vi "Load Player Types.vi"(8 "error in":errorcluster, 11 "Reversi in":refnum<class "Reversi.lvclass">) -> (0 "error out":errorcluster, 3 "Reversi out":refnum<class "Reversi.lvclass">)   [LabVIEW 2020, in "Reversi.lvlib" / "Reversi.lvclass"]
uses:
  Reversi.lvclass
  Player/Player.lvclass
  Reversi.lvclass/Reversi.ctl
  NonOOPlayer/NonOOPlayer.lvclass
  J:/Code/Reversi/Reversi/Player/Player.lvclass
  Human/Human.lvclass
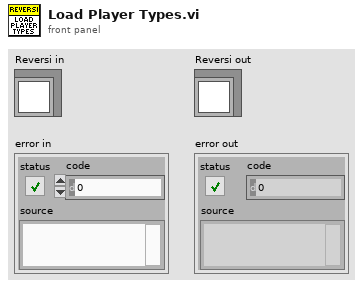
[diagram p1: front panel]
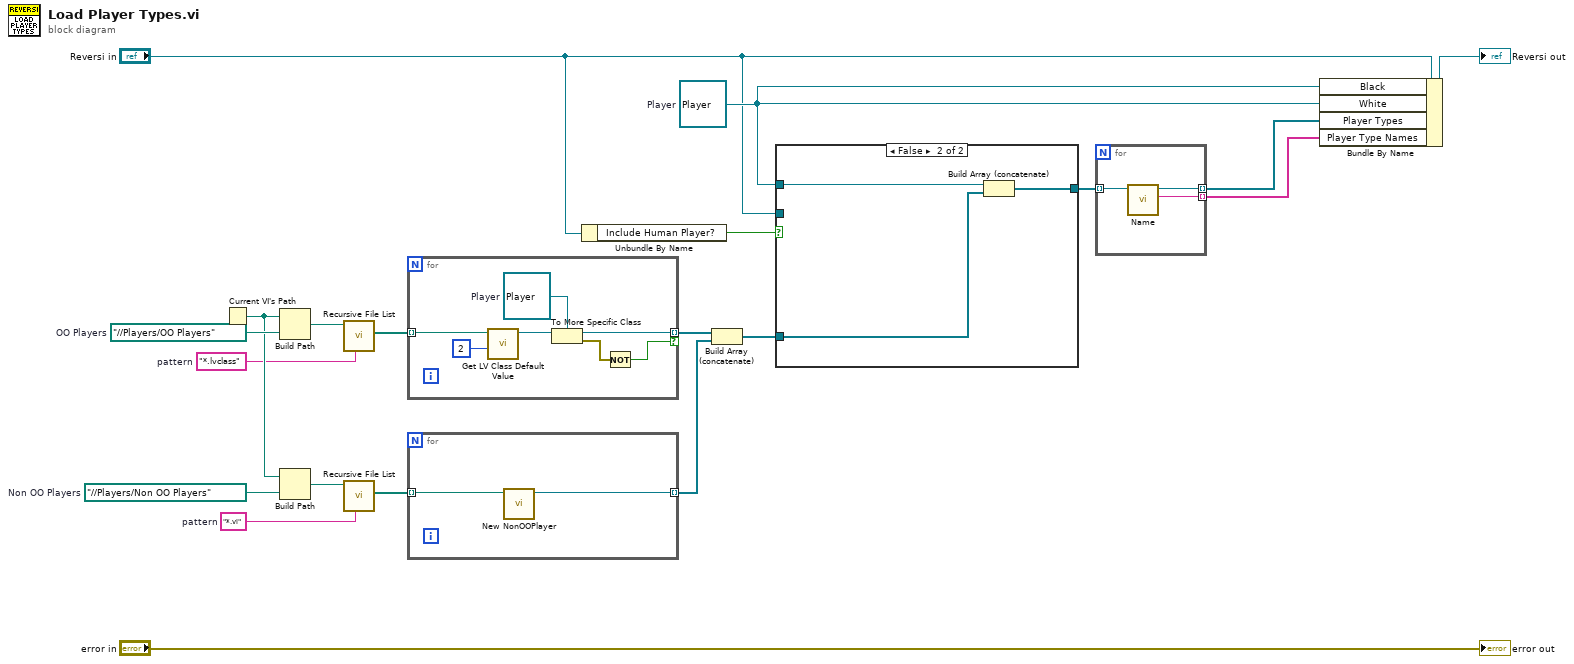
[diagram p0: block diagram]
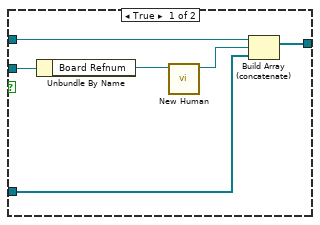
[diagram p2: hidden frame]
diagram:
  w9 = "*.vi"  # pattern
  w10 = "*.lvclass"  # pattern
  w13 = path "../../Players/Non OO Players"  # Non OO Players
  w14 = path "../../Players/OO Players"  # OO Players
  w17 = refnum<class "Player.lvclass"> refnum  # Player
  n1 = Current VI's Path() -> (path=w12:path)
  n2 = Build Path(base path=w12, name or relative path=w14) -> (appended path=w11:path)
  n3 = Build Path(base path=w12, name or relative path=w13) -> (appended path=w8:path)
  n4 = call <vilib>:"Recursive File List.vi"("pattern"=w10, "Folder Path"=w11) -> ("All Files in Dir"=w7:path[])  [unwired: 5 in, 4 out]
  n5 = call <vilib>:"Recursive File List.vi"("pattern"=w9, "Folder Path"=w8) -> ("All Files in Dir"=w6:path[])  [unwired: 5 in, 4 out]
  n6 = for {
    tunnel: w7 -> [w26] mode=indexing
    tunnel: [w22] -> w5 mode=indexing if=w21
    w23 = refnum<class "Player.lvclass"> refnum  # Player
    n7 = call <vilib>:"Get LV Class Default Value.vi"("options"=u32 2, "class path"=w26) -> ("object"=w24:refnum<class>)  [unwired: 8 in, 1 out]
    n8 = To More Specific Class(target class=w23, reference=w24) -> (specific class reference=w22:refnum<class "Player.lvclass">, error out=w27:errorcluster)  [unwired: 1 in]
    n9 = Not(x=w27) -> (.not. x?=w21:bool)
  }
  n10 = for {
    tunnel: w6 -> [w29] mode=indexing
    tunnel: [w28] -> w4 mode=indexing
    n11 = call "New NonOOPlayer.vi"("PlayerFilePath"=w29) -> ("NonOOPlayer out"=w28:refnum<class "NonOOPlayer.lvclass">)  [unwired: 9 in, 1 out]
  }
  n12 = Unbundle By Name("Reversi in") -> ("Include Human Player?"=w1:bool)
  n13 = Build Array (concatenate)(w5, w4) -> (w3:refnum<class "Player.lvclass">[])
  n14 = case shown="False" w1 {
    tunnel: [w35 w38] -> w19
    tunnel: w17 -> [w34 w37]
    tunnel: w3 -> [w33 w36]
    tunnel: "Reversi in" -> [w31 _]
    frame True {
      n15 = Unbundle By Name(w31) -> ("Board Refnum"=w32:refnum<vi>)
      n16 = call "New Human.vi"("Board Refnum"=w32) -> ("Human out"=w30:refnum<class "Human.lvclass">)  [unwired: 9 in, 1 out]
      n17 = Build Array (concatenate)(w34, w30, w33) -> (w35:refnum<class "Player.lvclass">[])
    }
    frame False {
      n18 = Build Array (concatenate)(w37, w36) -> (w38:refnum<class "Player.lvclass">[])
    }
  }
  n19 = for {
    tunnel: w19 -> [w41] mode=indexing
    tunnel: [w40] -> w16 mode=indexing
    tunnel: [w39] -> w15 mode=indexing
    n20 = call-dynamic "Name.vi"("Player in"=w41) -> ("Name"=w39:string, "Player out"=w40:refnum<class "Player.lvclass">)  [unwired: 8 in, 1 out]
  }
  n21 = Bundle By Name(cluster="Reversi in", "Black"=w17, "White"=w17, "Player Types"=w16, "Player Type Names"=w15) -> (→"Reversi out":refnum<class "Reversi.lvclass">)
  "error out" <- "error in"
